vi "Permutation.vi"(1 "array":bool[](array[boolean])) -> (0 "Array":bool[](array[boolean]))   [LabVIEW 2013]
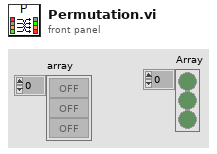
[diagram p1: front panel]
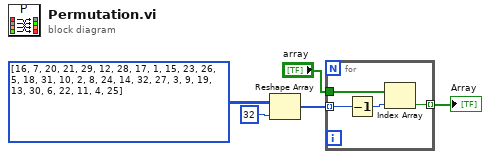
[diagram p0: block diagram]
diagram:
  n1 = Reshape Array(u8[][] [[16, 7, 20, 21, 29, 12, 28, 17], [1, 15, 23, 26, 5, 18, 31, 10], [2, 8, 24, 14, 32, 27, 3, 9], [19, 13, 30, 6, 22, 11, 4, 25]], 32 ("dimension size")) -> (w4:u8[])
  n2 = for {
    tunnel: "array" -> [w8]
    tunnel: w4 -> [w9] mode=indexing
    tunnel: [w6] -> w1 mode=indexing
    n3 = Decrement(x=w9) -> (x-1=w7:u8)
    n4 = Index Array(array=w8, index=w7) -> (element=w6:bool)
  }
  "Array" <- w1
